vi "everest_adc_bias_init.vi"(8 "error in":errorcluster, 11 "VISA resource name":refnum<visa-resource-name>="COM3") -> (0 "error out":errorcluster)   [LabVIEW 2015]
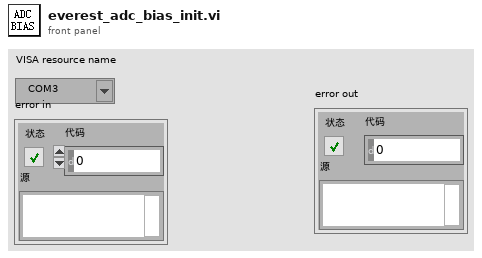
[diagram p1: front panel]
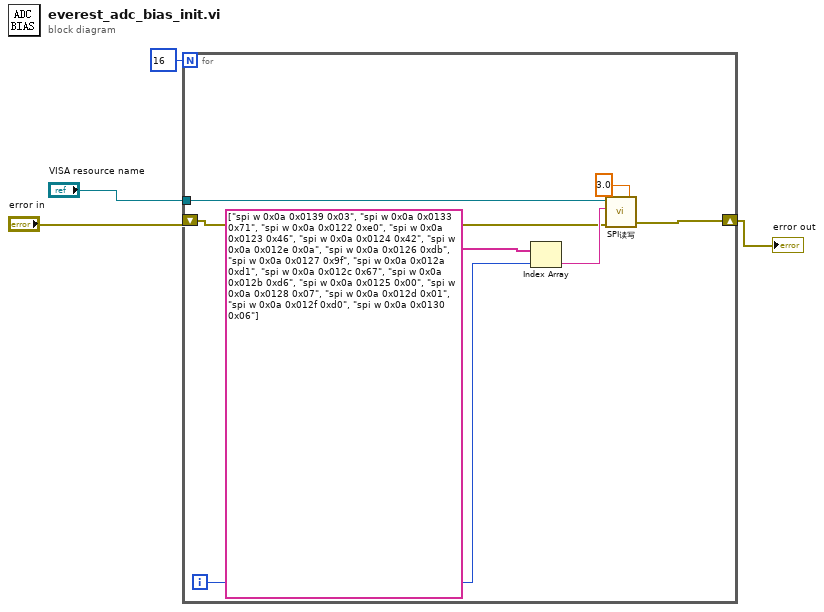
[diagram p0: block diagram]
diagram:
  n1 = for {
    N: 16 -> [_]
    shift-right: [w7] -> w4
    shift-left: "error in" -> [w8]
    tunnel: "VISA resource name" -> [w6]
    i -> [w10]
    n2 = Index Array(array=string[] ["spi w 0x0a 0x0139 0x03", "spi w 0x0a 0x0133 0x71", "spi w 0x0a 0x0122 0xe0", "spi w 0x0a 0x0123 0x46", "spi w 0x0a 0x0124 0x42", "spi w 0x0a 0x012e 0x0a", "spi w 0x0a 0x0126 0xdb", "spi w 0x0a 0x0127 0x9f", "spi w 0x0a 0x012a 0xd1", "spi w 0x0a 0x012c 0x67", "spi w 0x0a 0x012b 0xd6", "spi w 0x0a 0x0125 0x00", "spi w 0x0a 0x0128 0x07", "spi w 0x0a 0x012d 0x01", "spi w 0x0a 0x012f 0xd0", "spi w 0x0a 0x0130 0x06"], index=w10) -> (element=w9:string)
    n3 = call "SPI读写.vi"("DELAY"=3.0, "error in (no error)"=w8, "往芯片写数据"=w9, "VISA resource name"=w6) -> ("error out"=w7:errorcluster)  [unwired: 1 in, 1 out]
  }
  "error out" <- w4
